vi "Atto DRY Interface get Attodry Error Message.vi"(8 "error in (no error)":errorcluster, 10 "len":i32, 11 "ErrorMessage":string) -> (0 "error out":errorcluster, 2 "function return":i32, 3 "ErrorMessage out":string)   [LabVIEW 2016, in "attoDRYLib.lvlib"]
doc: "int32_t __cdecl AttoDRY_Interface_getAttodryErrorMessage(char ErrorMessage[], \n int32_t len);"
uses:
  <userlib>/attoDRYLib/attoDRYLib.lvlib
  <userlib>/attoDRYLib/attoDRYLib.dll
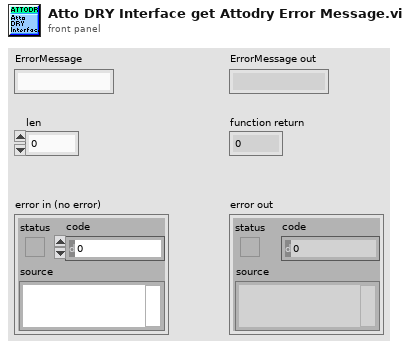
[diagram p1: front panel]
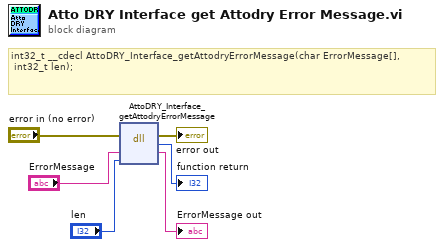
[diagram p0: block diagram]
diagram:
  # "int32_t __cdecl AttoDRY_Interface_getAttodryErrorMessage(char ErrorMessage[], \n\tint32_t len);"
  n1 = dll-call lib="C:/Program Files (x86)/National Instruments/LabVIEW 2016/user.lib/attoDRYLib/attoDRYLib.*" fn="AttoDRY_Interface_getAttodryErrorMessage"(error in="error in (no error)", "ErrorMessage"="ErrorMessage", "len"="len") -> (error out=→"error out":errorcluster, →"function return":i32, "ErrorMessage"=→"ErrorMessage out":string)  [unwired: 3 in, 1 out]
